vi "Check number input.vi"(10 "numberStr":string) -> (2 "valid":bool)   [LabVIEW 2018]
uses:
  <vilib>/regexp/Match Regular Expression.xnode
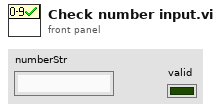
[diagram p1: front panel]
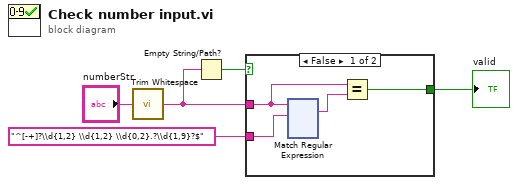
[diagram p0: block diagram]
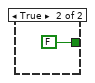
[diagram p2: hidden frame]
diagram:
  n1 = call <vilib>:"Trim Whitespace.vi"("string"="numberStr") -> ("trimmed string"=w4:string)  [unwired: 1 in]
  n2 = Empty String/Path?(string/path=w4) -> (empty?=w2:bool)
  n3 = case shown="False" w2 {
    tunnel: w4 -> [w8 _]
    tunnel: "^[-+]?\\d{1,2} \\d{1,2} \\d{0,2}.?\\d{1,9}?$" ("Regular Expression") -> [w9 _]
    tunnel: [w6 FALSE] -> w1
    frame False {
      n4 = xnode "Match Regular Expression"("input string"=w8, "regular expression"=w9) -> ("whole match"=w7:string)  [unwired: 4 in, 4 out]
      n5 = Equal?(x=w8, y=w7) -> (x = y?=w6:bool)
    }
    frame True {
    }
  }
  "valid" <- w1
